vi "DataPacker_BundleQueueItems.vi"(8 "error in (no error)":errorcluster, 11 "DataPacker in":refnum<class "DataPacker.lvclass">) -> (0 "error out":errorcluster, 2 "# elements in queue":i32, 3 "DataPacker out":refnum<class "DataPacker.lvclass">)   [LabVIEW 2018, in "DataPacker.lvclass"]
uses:
  DataPacker.lvclass
  DataPacker.lvclass/DataPacker.ctl
  DataStructures/GEM_BANK_ARRAY.lvclass/GEM_BANK_ARRAY.ctl
  DataStructures/GEM_BANK_ARRAY.lvclass
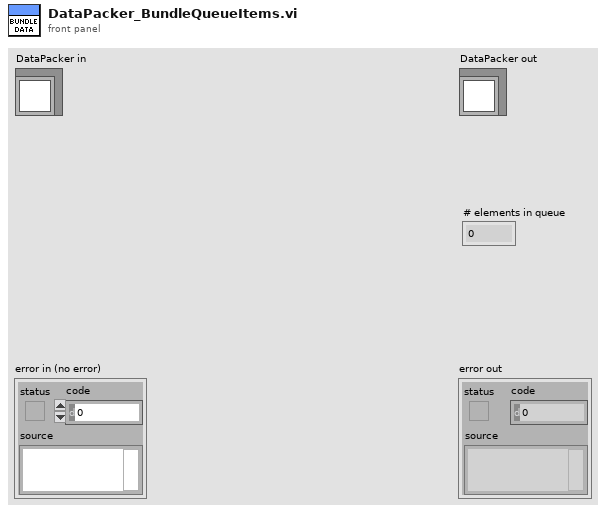
[diagram p1: front panel]
types:
  T1 = typedef "GEM_BANK_CLUSTER_typedef.ctl" = cluster{"Category":string, "Variable Name":string, "Equipment description":string, "History Settings":u16, "Period to update history plots":u16, "GEM_DATA Cluster":T2}
  T2 = typedef "GEM_DATA_cluster_typedef.ctl" = cluster{"DataType":string, "Formatted Data":u8[], "data byte order (Little Endian prefered)":enum16{"big-endian, network order", "native, host order", "little-endian"}}
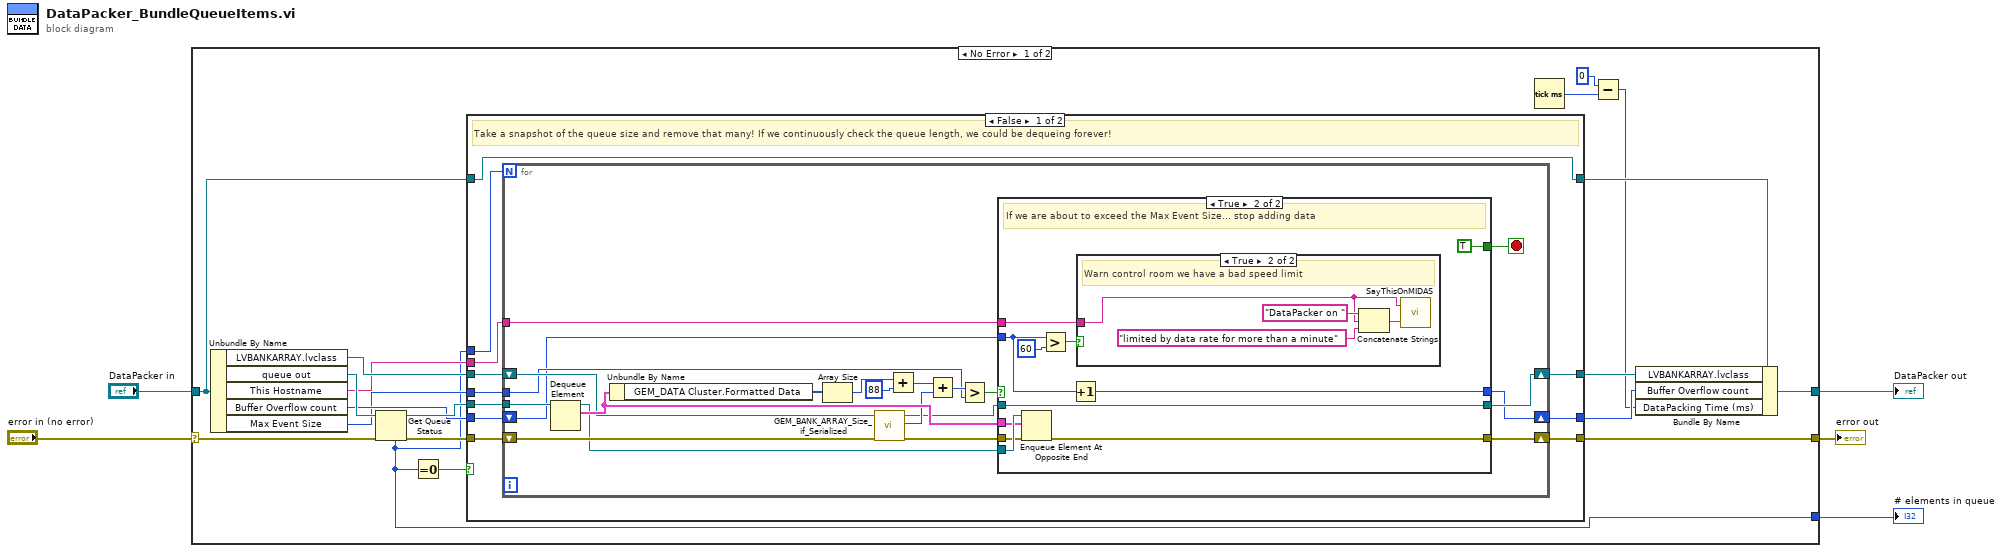
[diagram p0: block diagram]
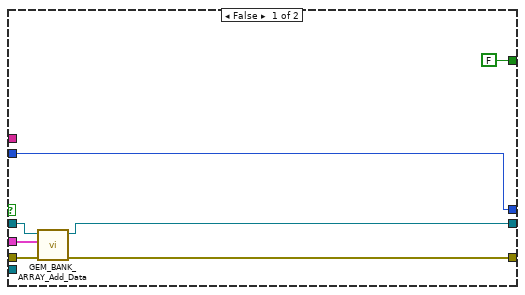
[diagram p2: hidden frame]
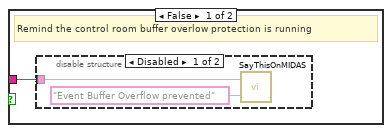
[diagram p3: hidden frame]
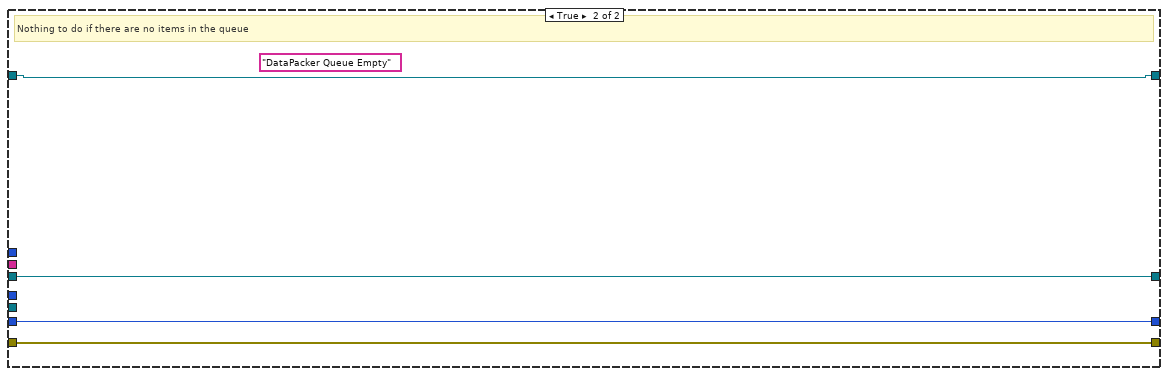
[diagram p5: hidden frame]
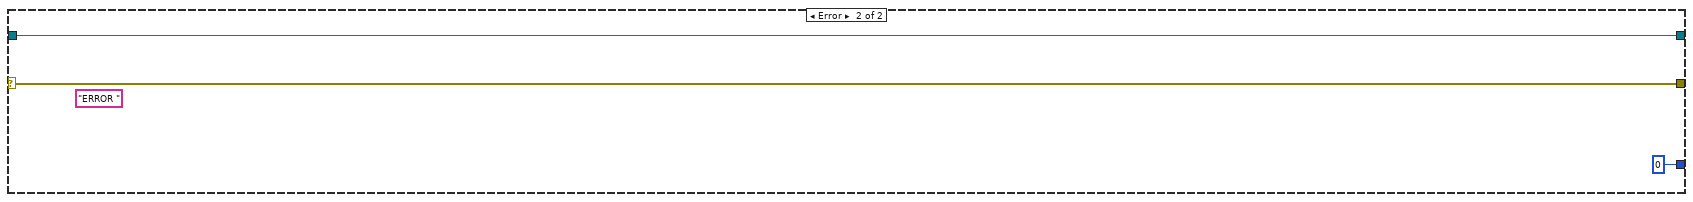
[diagram p6: hidden frame]
diagram:
  n1 = case shown="No Error" "error in (no error)" {
    selector: "error in (no error)" -> [w18 w88]
    tunnel: [w16 w88] -> w4
    tunnel: [w23 w87] -> w2
    tunnel: "DataPacker in" -> [w24 w87]
    tunnel: [w9 0 ("# elements in queue")] -> w1
    frame No Error {
      n2 = Unbundle By Name(w24) -> ("LVBANKARRAY.lvclass"=w17:refnum<class "GEM_BANK_ARRAY.lvclass">, "queue out"=w19:refnum<queue>, "This Hostname"=w11:string, "Buffer Overflow count"=w13:u32, "Max Event Size"=w10:u32)
      n3 = Get Queue Status(queue=w19, error in (no error)=w18) -> (queue out=w21:refnum<queue>, error out=w22:errorcluster, # elements in queue=w9:i32)  [unwired: 1 in, 5 out]
      n4 = Equal To 0?(x=w9) -> (x = 0?=w20:bool)
      n5 = case shown="False" w20 {
        tunnel: w9 -> [w34 _]
        tunnel: w21 -> [w33 _]
        tunnel: w22 -> [w31 w85]
        tunnel: w17 -> [w32 w84]
        tunnel: [w25 w85] -> w16
        tunnel: [w27 w84] -> w15
        tunnel: w24 -> [w35 w83]
        tunnel: [w35 w83] -> w14
        tunnel: w13 -> [w29 w82]
        tunnel: [w26 w82] -> w12
        tunnel: w11 -> [w28 _]
        tunnel: w10 -> [w30 _]
        frame False {
          # "Take a snapshot of the queue size and remove that many! If we continuously check the queue length, we could be dequeing forever!"
          n6 = for {
            N: w34 -> [_]
            tunnel: w33 -> [w56]
            shift-right: [w55] -> w27
            shift-left: w32 -> [w51]
            shift-right: [w54] -> w25
            shift-left: w31 -> [w49]
            tunnel: w30 -> [w47]
            shift-right: [w40] -> w26
            shift-left: w29 -> [w41]
            tunnel: w28 -> [w39]
            stop <- w42 stop-if-true
            n7 = Dequeue Element(queue=w56) -> (queue out=w43:refnum<queue>, element=w53:T1)  [unwired: 2 in, 2 out]
            n8 = Unbundle By Name(w53) -> ("GEM_DATA Cluster.Formatted Data"=w52:u8[])
            n9 = Array Size(array=w52) -> (size(s)=w38:i32)
            n10 = call "GEM_BANK_ARRAY_Size_if_Serialized.vi"("error in (no error)"=w49, "GEM_BANK_ARRAY in"=w51) -> ("error out"=w45:errorcluster, "Size if Serialized"=w50:u32, "GEM_BANK_ARRAY out"=w44:refnum<class "GEM_BANK_ARRAY.lvclass">)  [unwired: 7 in]
            n11 = Add(x=w38, y=88) -> (x+y=w36:i32)
            n12 = Add(x=w36, y=w50) -> (x+y=w48:u32)
            n13 = Greater?(x=w48, y=w47) -> (0:w46:bool)
            n14 = case shown="True" w46 {
              tunnel: [w63 w69] -> w55
              tunnel: [w60 w71] -> w54
              tunnel: w53 -> [w62 w73]
              tunnel: w45 -> [w61 w72]
              tunnel: w44 -> [w59 w69]
              tunnel: w43 -> [_ w74]
              tunnel: [FALSE TRUE] -> w42
              tunnel: w41 -> [w57 w66]
              tunnel: [w57 w68] -> w40
              tunnel: w39 -> [_ w67]
              frame False {
                n15 = call "GEM_BANK_ARRAY_Add_Data.vi"("error in (no error)"=w61, "GEM BANK Cluster"=w62, "LVBANKARRAY in"=w59) -> ("error out"=w60:errorcluster, "LVBANKARRAY out"=w63:refnum<class "GEM_BANK_ARRAY.lvclass">)  [unwired: 7 in]
              }
              frame True {
                # "If we are about to exceed the Max Event Size... stop adding data"
                n16 = Enqueue Element At Opposite End(queue=w74, element=w73, error in (no error)=w72) -> (error out=w71:errorcluster)  [unwired: 1 in, 2 out]
                n17 = Greater?(x=w66, y=u32 60) -> (0:w64:bool)
                n18 = Increment(x=w66) -> (x+1=w68:u32)
                n19 = case shown="True" w64 {
                  tunnel: w67 -> [w75 w80]
                  frame False {
                    # "Remind the control room buffer overlow protection is running"
                    n20 = disable-structure shown="Disabled" {
                      disable-tunnel: w75 -> [w76 _]
                      frame Disabled {
                        n21 = call "SayThisOnMIDAS.vi"("String"="Event Buffer Overflow prevented", "Hostname (Optional)"=w76) -> ()  [unwired: 1 out]
                      }
                      frame Enabled {
                      }
                    }
                  }
                  frame True {
                    # "Warn control room we have a bad speed limit"
                    n22 = Concatenate Strings("DataPacker on " ("string"), w80, "limited by data rate for more than a minute" ("String")) -> (w78:string)
                    n23 = call "SayThisOnMIDAS.vi"("String"=w78, "Hostname (Optional)"=w80) -> ()  [unwired: 1 out]
                  }
                }
              }
            }
          }
        }
        frame True {
          (unwired) "DataPacker Queue Empty" ("MIDAS Reply")
          # "Nothing to do if there are no items in the queue"
        }
      }
      n24 = Tick Count (ms)() -> (millisecond timer value=w8:u32)
      n25 = Subtract(x=u32 0, y=w8) -> (x-y=w6:u32)
      n26 = Bundle By Name(cluster=w14, "LVBANKARRAY.lvclass"=w15, "Buffer Overflow count"=w12, "DataPacking Time (ms)"=w6) -> (w23:refnum<class "DataPacker.lvclass">)
    }
    frame Error {
      (unwired) "ERROR " ("MIDAS Reply")
    }
  }
  "error out" <- w4
  "DataPacker out" <- w2
  "# elements in queue" <- w1
